vi "Stop&off.vi"(0 "Laser GPIB":u8=10 max=100, 1 "Motor GPIB":string="6") -> ()   [LabVIEW 2010]
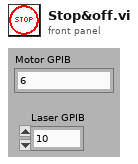
[diagram p1: front panel]
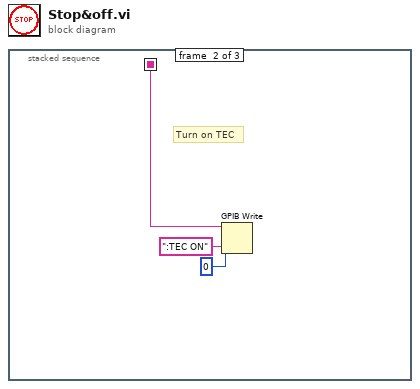
[diagram p0: block diagram]
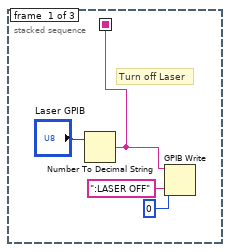
[diagram p2: hidden frame]
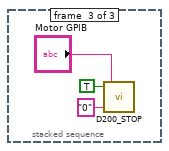
[diagram p3: hidden frame]
diagram:
  n1 = stacked-sequence {
    seq-local: [w1 _ _] -> [_ w5 _]
    frame #0 {
      # "Turn off Laser"
      n2 = Number To Decimal String(number="Laser GPIB") -> (decimal integer string=w1:string)  [unwired: 1 in]
      n3 = GPIB Write(0:w1, 1:":LASER OFF" ("data"), 2:i16 0 ("mode (0)")) -> ()  [unwired: 2 in, 2 out]
    }
    frame #1 {
      # "Turn on TEC"
      n4 = GPIB Write(0:w5, 1:":TEC ON" ("data"), 2:i16 0 ("mode (0)")) -> ()  [unwired: 2 in, 2 out]
    }
    frame #2 {
      n5 = call "D200_STOP.vi"("Stoptype"="0", "GPIB Addr"="Motor GPIB", "Permission"=TRUE) -> ()  [unwired: 1 out]
    }
  }
